vi "例程07-中级计算器(wait finish).vi"() -> ()   [LabVIEW 2018]
panel:
  in  "操作临时存储":string
  in  "输入临时存储":string
  in  "过程显示界面":string
  in  "结果":string
  in  "输入2":string
  in  "输入1":string
  in  "等于":bool
  in  "清除":bool
  in  "/":bool
  in  "小数点":bool
  in  "数字0":bool
  in  "正负号":bool
  in  "*":bool
  in  "-":bool
  in  "+":bool
  in  "数字9":bool
  in  "数字8":bool
  in  "数字7":bool
  in  "数字6":bool
  in  "数字5":bool
  in  "数字4":bool
  in  "数字3":bool
  in  "数字2":bool
  in  "数字1":bool
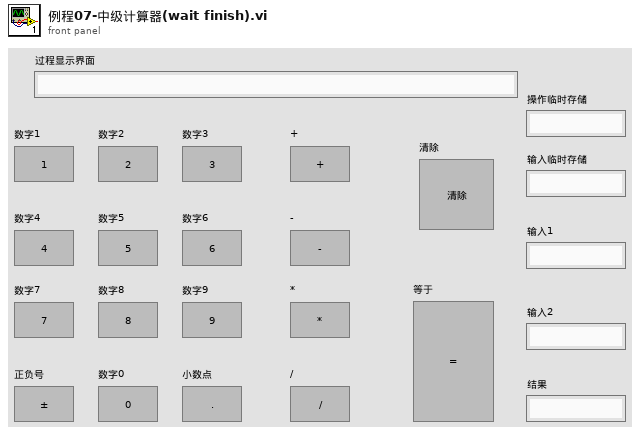
[diagram p1: front panel]
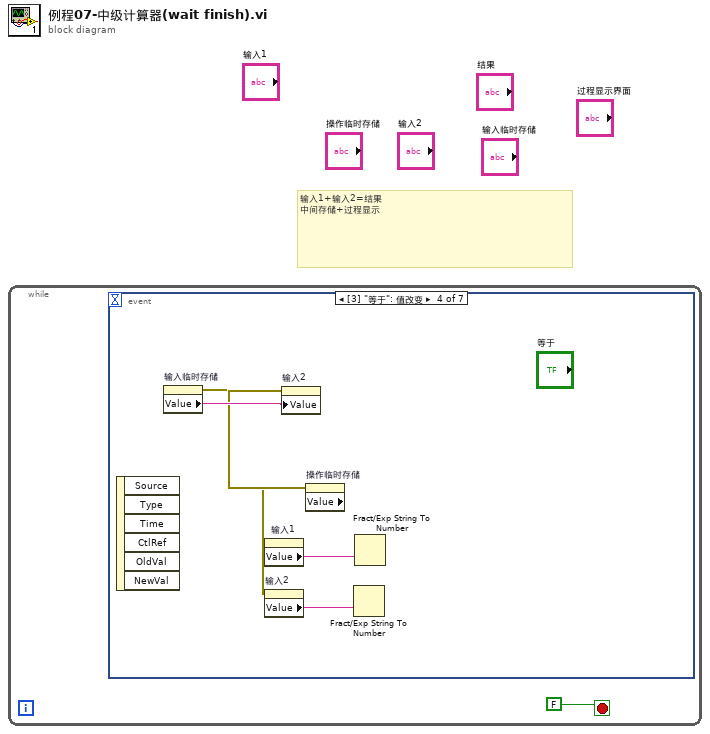
[diagram p0: block diagram]
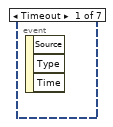
[diagram p2: hidden frame]
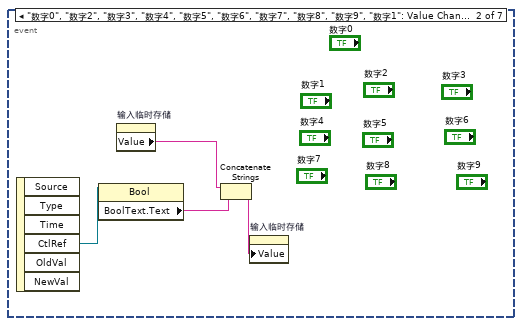
[diagram p3: hidden frame]
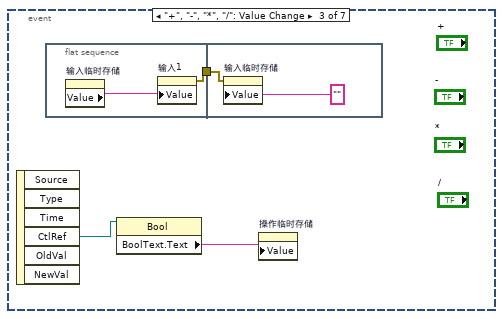
[diagram p4: hidden frame]
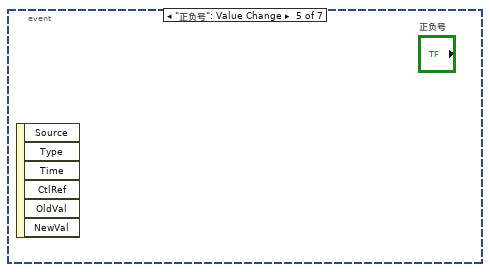
[diagram p5: hidden frame]
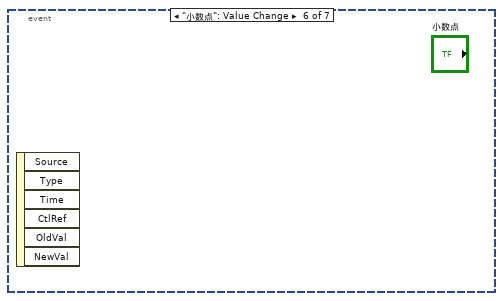
[diagram p6: hidden frame]
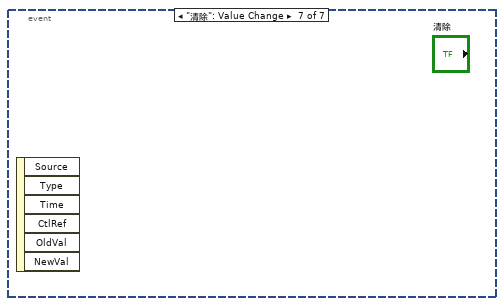
[diagram p7: hidden frame]
diagram:
  # "输入1+输入2=结果\n中间存储+过程显示"
  n1 = while {
    stop <- FALSE stop-if-true
    n2 = event shown="[3] \"等于\": 值改变" {
      selector: _ -> [_ _ _ _ _ _ _]
      dyn-events: _ -> [_ _ _ _ _ _ _]
      timeout: _ -> [_ _ _ _ _ _ _]
      event Timeout {
        n3 = event-data() -> ()  [unwired: 1 in, 3 out]
      }
      event "数字0", "数字2", "数字3", "数字4", "数字5", "数字6", "数字7", "数字8", "数字9", "数字1": Value Change {
        n4 = event-data() -> ("CtlRef"=w5:refnum<vi>)  [unwired: 1 in, 5 out]
        n5 = property class="Bool"(reference=w5) -> ("BoolText.Text"=w2:string)  [unwired: 1 in, 2 out]
        n6 = property on="输入临时存储" class="Str"() -> ("Value"=w3:string)  [unwired: 2 in, 2 out]
        n7 = Concatenate Strings(w3, w2) -> (w4:string)
        n8 = property on="输入临时存储" class="Str"("Value"=w4) -> ()  [unwired: 2 in, 2 out]
      }
      event "+", "-", "*", "/": Value Change {
        n9 = event-data() -> ("CtlRef"=w8:refnum<vi>)  [unwired: 1 in, 5 out]
        n10 = flat-sequence {
          tunnel: [w9] -> w6
          tunnel: w6 -> [w11]
          frame #0 {
            n11 = property on="输入临时存储" class="Str"() -> ("Value"=w10:string)  [unwired: 2 in, 2 out]
            n12 = property on="输入1" class="Str"("Value"=w10) -> (error out=w9:errorcluster)  [unwired: 2 in, 1 out]
          }
          frame #1 {
            n13 = property on="输入临时存储" class="Str"(error in=w11, "Value"="" ("输入临时存储")) -> ()  [unwired: 1 in, 2 out]
          }
        }
        n14 = property class="Bool"(reference=w8) -> ("BoolText.Text"=w7:string)  [unwired: 1 in, 2 out]
        n15 = property on="操作临时存储" class="Str"("Value"=w7) -> ()  [unwired: 2 in, 2 out]
      }
      event "等于": Value Change {
        n16 = event-data() -> ()  [unwired: 1 in, 6 out]
        n17 = property on="输入临时存储" class="Str"() -> (error out=w13:errorcluster, "Value"=w18:string)  [unwired: 2 in, 1 out]
        n18 = property on="输入1" class="Str"() -> ("Value"=w16:string)  [unwired: 2 in, 2 out]
        n19 = property on="输入2" class="Str"(error in=w13, "Value"=w18) -> (error out=w17:errorcluster)  [unwired: 1 in, 1 out]
        n20 = property on="操作临时存储" class="Str" props=["Value"](error in=w17) -> (error out=w14:errorcluster)  [unwired: 1 in, 2 out]
        n21 = property on="输入2" class="Str"(error in=w14) -> ("Value"=w15:string)  [unwired: 1 in, 2 out]
        n22 = Fract/Exp String To Number(string=w15) -> ()  [unwired: 3 in, 2 out]
        n23 = Fract/Exp String To Number(string=w16) -> ()  [unwired: 3 in, 2 out]
      }
      event "正负号": Value Change {
        n24 = event-data() -> ()  [unwired: 1 in, 6 out]
      }
      event "小数点": Value Change {
        n25 = event-data() -> ()  [unwired: 1 in, 6 out]
      }
      event "清除": Value Change {
        n26 = event-data() -> ()  [unwired: 1 in, 6 out]
      }
    }
  }
